vi "xml_get_targets.vi"(0 "XML Path":path=path "D:/Test Management/Farmer/XML/targets.xml", 1 "error in (no error)":errorcluster) -> (2 "Target Array":T2(array[cluster]), 3 "success?":bool, 4 "error out":errorcluster)   [LabVIEW 2011]
uses:
  TargetData.ctl
  <vilib>/xml/Load XML File.vi
  <vilib>/xml/Close Reference(Node).vi
  <vilib>/xml/NI_XML.lvlib
  Program Files/National Instruments/LabVIEW 2011/resource/objmgr/DOMUserDefRef.rc
panel:
  in  "Target Array Type":T2(array[cluster])
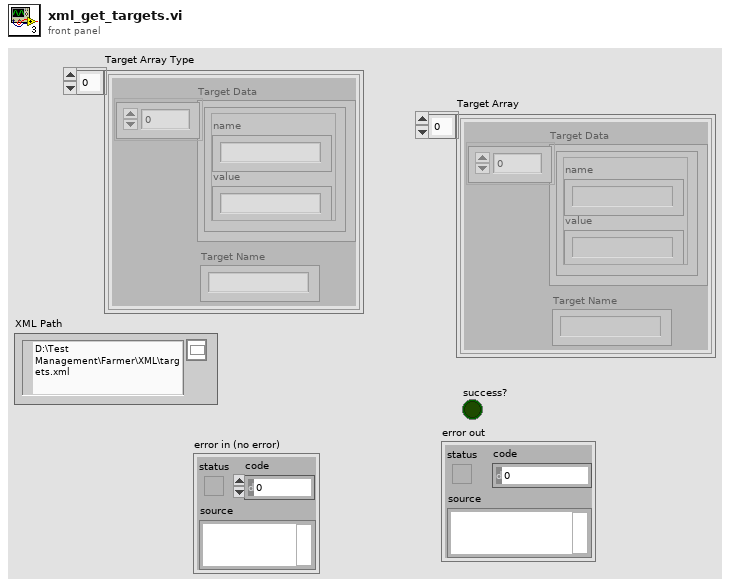
[diagram p1: front panel]
types:
  T1 = typedef "TargetData.ctl" = cluster{"name":string, "value":string}[]
  T2 = cluster{"Target Data":T1, "Target Name":string}[]
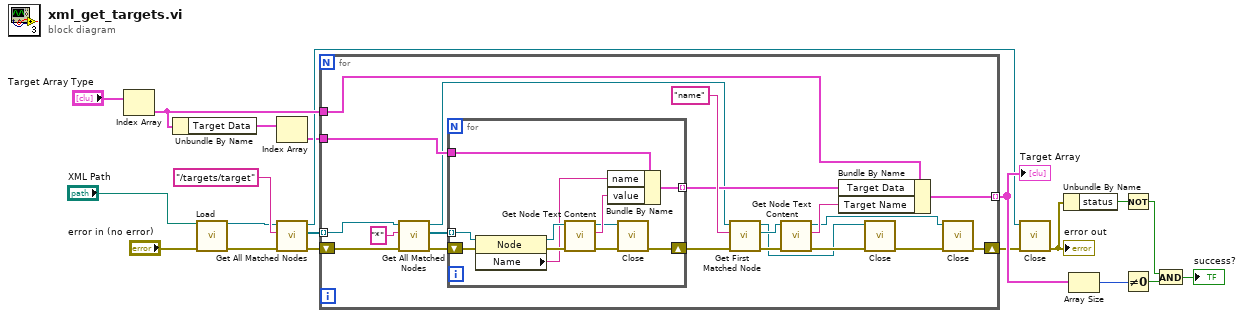
[diagram p0: block diagram]
diagram:
  n1 = Index Array(array="Target Array Type") -> (element=w12:cluster{"Target Data":T1, "Target Name":string})  [unwired: 1 in]
  n2 = Unbundle By Name(w12) -> ("Target Data"=w3:T1)
  n3 = call-poly <vilib>:"Load.vi"("path to XML document"="XML Path", "error in (no error)"="error in (no error)") -> ("DOM document out"=w5:refnum<k20>, "error out"=w20:errorcluster)  [unwired: 11 in, 1 out]
  n4 = Index Array(array=w3) -> (element=w2:cluster{"name":string, "value":string})  [unwired: 1 in]
  n5 = call <vilib>:"Get All Matched Nodes.vi"("error in (no error)"=w20, "XPath expression"="/targets/target", "node in"=w5) -> ("error out"=w19:errorcluster, "node result array"=w14:refnum<k20>[], "node out"=w4:refnum<k20>)  [unwired: 6 in]
  n6 = for {
    tunnel: w14 -> [w36] mode=indexing
    tunnel: w2 -> [w35]
    tunnel: w12 -> [w34]
    shift-right: [w22] -> w6
    shift-left: w19 -> [w40]
    tunnel: [w27] -> w11 mode=indexing
    n7 = call <vilib>:"Get All Matched Nodes.vi"("error in (no error)"=w40, "XPath expression"="*", "node in"=w36) -> ("error out"=w37:errorcluster, "node result array"=w38:refnum<k20>[], "node out"=w26:refnum<k20>)  [unwired: 6 in]
    n8 = for {
      tunnel: w38 -> [w51] mode=indexing
      shift-right: [w43] -> w33
      shift-left: w37 -> [w49]
      tunnel: [w47] -> w29 mode=indexing
      tunnel: w35 -> [w41]
      n9 = property class="Node"(reference=w51, error in=w49) -> (reference out=w50:refnum<k20>, error out=w48:errorcluster, "Name"=w46:string)
      n10 = call <vilib>:"Get Node Text Content.vi"("error in (no error)"=w48, "node in"=w50) -> ("error out"=w44:errorcluster, "node text"=w45:string, "node out"=w42:refnum<k20>)  [unwired: 7 in]
      n11 = Bundle By Name(cluster=w41, "name"=w46, "value"=w45) -> (w47:cluster{"name":string, "value":string})
      n12 = call-poly <vilib>:"Close.vi"("error in (no error)"=w44, "node"=w42) -> ("error out"=w43:errorcluster)  [unwired: 7 in]
    }
    n13 = call <vilib>:"Get First Matched Node.vi"("error in (no error)"=w33, "XPath expression"="name", "node in"=w26) -> ("error out"=w28:errorcluster, "node result"=w31:refnum<k20>, "node out"=w24:refnum<k20>)  [unwired: 6 in]
    n14 = call <vilib>:"Get Node Text Content.vi"("error in (no error)"=w28, "node in"=w31) -> ("error out"=w25:errorcluster, "node text"=w30:string, "node out"=w21:refnum<k20>)  [unwired: 7 in]
    n15 = Bundle By Name(cluster=w34, "Target Data"=w29, "Target Name"=w30) -> (w27:cluster{"Target Data":T1, "Target Name":string})
    n16 = call-poly <vilib>:"Close.vi"("error in (no error)"=w25, "node"=w24) -> ("error out"=w23:errorcluster)  [unwired: 7 in]
    n17 = call-poly <vilib>:"Close.vi"("error in (no error)"=w23, "node"=w21) -> ("error out"=w22:errorcluster)  [unwired: 7 in]
  }
  "Target Array" <- w11
  n18 = call-poly <vilib>:"Close.vi"("error in (no error)"=w6, "node"=w4) -> ("error out"=w17:errorcluster)  [unwired: 7 in]
  "error out" <- w17
  n19 = Unbundle By Name(w17) -> ("status"=w16:bool)
  n20 = Array Size(array=w11) -> (size(s)=w10:i32)
  n21 = Not(x=w16) -> (.not. x?=w9:bool)
  n22 = Not Equal To 0?(x=w10) -> (x != 0?=w8:bool)
  n23 = And(x=w9, y=w8) -> (x .and. y?=→"success?":bool)
